vi "dvp Vi Set Contrast.vi"(10 "Contrast":i32, 11 "handle":u32) -> (3 "function return":u32(ring))   [LabVIEW 2018, in "LabViewDVPCamera.lvlib"]
doc: "LabviewDvp2Api dvpStatus dvpViSetContrast(dvpHandle handle, dvpInt32 Contrast);"
uses:
  LabViewDVPCamera.lvlib
  LabViewDVPCamera/LabViewDVPCamera.dll
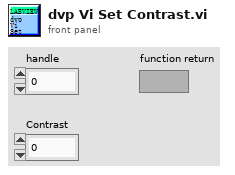
[diagram p1: front panel]
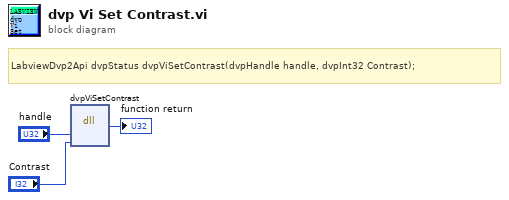
[diagram p0: block diagram]
diagram:
  # "LabviewDvp2Api dvpStatus dvpViSetContrast(dvpHandle handle, dvpInt32 Contrast);"
  n1 = dll-call lib="C:/Program Files (x86)/DVP2 Labview cn 64/Sample/LabViewDVPCamera/LabViewDVPCamera.*" fn="dvpViSetContrast"("handle"="handle", "Contrast"="Contrast") -> (→"function return":u32)  [unwired: 5 in, 2 out]
